vi "Reading temperature (SILAR).vi"(8 "error in":errorcluster, 11 "Arduino Resource in":T1={"VISA resource"="", "Board Type"=enum."Uno", "Connection Type"=enum."USB / Serial", "Bytes Per Packet (15)"=15}) -> (0 "error out":errorcluster, 3 "Arduino Resource":T1={"VISA resource"="", "Board Type"=enum."Uno", "Connection Type"=enum."USB / Serial", "Bytes Per Packet (15)"=15}, 4 "read buffer":string)   [LabVIEW 2016]
uses:
  <vilib>/LabVIEW Interface for Arduino/Type Defs/Arduino Resource.ctl
  <vilib>/LabVIEW Interface for Arduino/Type Defs/Board Type.ctl
  <vilib>/LabVIEW Interface for Arduino/LabVIEW Interface for Arduino.lvlib
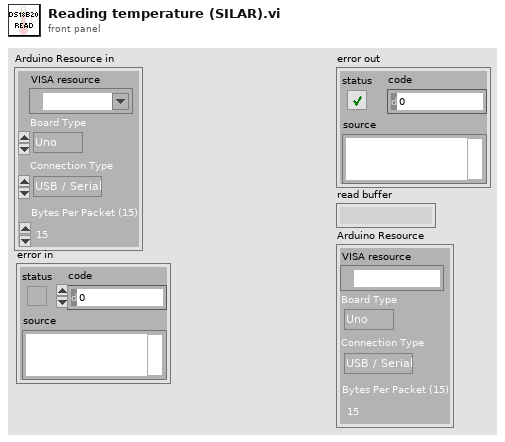
[diagram p1: front panel]
types:
  T1 = typedef "LabVIEW Interface for Arduino.lvlib/Arduino Resource.ctl" = cluster{"VISA resource":refnum<visa-resource-name>, "Board Type":T2, "Connection Type":enum8{"USB / Serial"}, "Bytes Per Packet (15)":u8}
  T2 = typedef "LabVIEW Interface for Arduino.lvlib/Board Type.ctl" = enum16{"Uno", "Dimuelanove w/Atmega 328", "Mega 2560"}
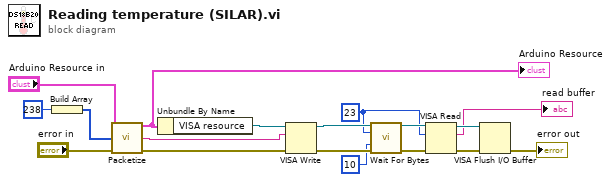
[diagram p0: block diagram]
diagram:
  w5 = u32 23 ("Bytes To Read")
  n1 = Build Array(238) -> (w15:i32[])
  n2 = call <vilib>:"Packetize.vi"("Arduino Resource"="Arduino Resource in", "Data"=w15, "error in"="error in") -> ("Arduino Resource"=w13:T1, "Packet"=w17:string, "error out"=w16:errorcluster)  [unwired: 10 in]
  "Arduino Resource" <- w13
  n3 = Unbundle By Name(w13) -> ("VISA resource"=w18:refnum<visa-resource-name>)
  n4 = VISA Write(VISA resource name=w18, write buffer=w17, error in (no error)=w16) -> (VISA resource name out=w9:refnum<visa-resource-name>, error out=w8:errorcluster)  [unwired: 1 out]
  n5 = call <vilib>:"Wait For Bytes.vi"("VISA resource"=w9, "Bytes To Read"=w5, "Time Out (100 ms)"=10, "error in"=w8) -> ("VISA resource"=w6:refnum<visa-resource-name>, "error out"=w7:errorcluster)  [unwired: 9 in, 1 out]
  n6 = VISA Read(VISA resource name=w6, byte count=w5, error in (no error)=w7) -> (VISA resource name out=w14:refnum<visa-resource-name>, read buffer=→"read buffer":string, error out=w11:errorcluster)  [unwired: 1 out]
  n7 = VISA Flush I/O Buffer(VISA resource name=w14, error in (no error)=w11) -> (error out=→"error out":errorcluster)  [unwired: 1 in, 1 out]
